vi "Create and Start gRPC Server.vi"(5 "Server Key File (.key)":path, 7 "Server Certificate File (.crt)":path, 8 "error in (no error)":errorcluster, 10 "Server Address":string="localhost:15882", 11 "Plugin Manager in":refnum<class "CIFPluginManager.lvclass">) -> (0 "error out":errorcluster, 3 "Plugin Manager out":refnum<class "CIFPluginManager.lvclass">)   [LabVIEW 2021, in "CIFPluginManager.lvclass"]
uses:
  CIFPluginManager.lvclass
  <vilib>/gRPC/LabVIEW gRPC Servicer/Servicer/Servicer.lvclass/Servicer.ctl
  CIFPluginManager.lvclass/CIFPluginManager.ctl
  <vilib>/gRPC/LabVIEW gRPC Servicer/Servicer/Servicer.lvclass
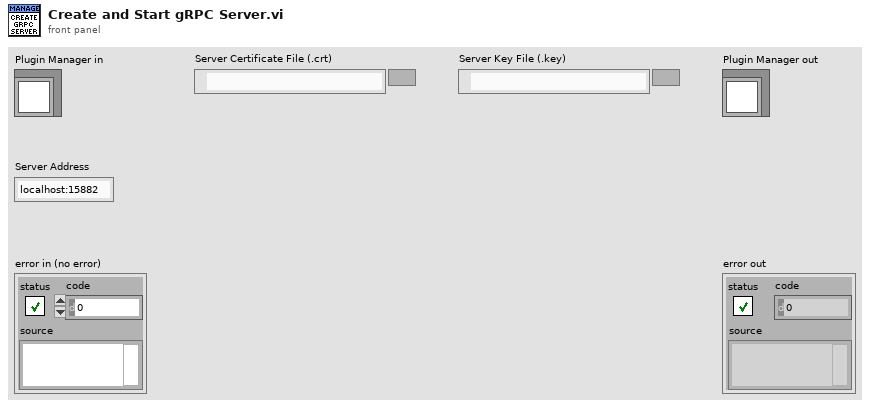
[diagram p1: front panel]
types:
  T1 = typedef "grpc-lvsupport-release.lvlib/grpcId.ctl" = u64
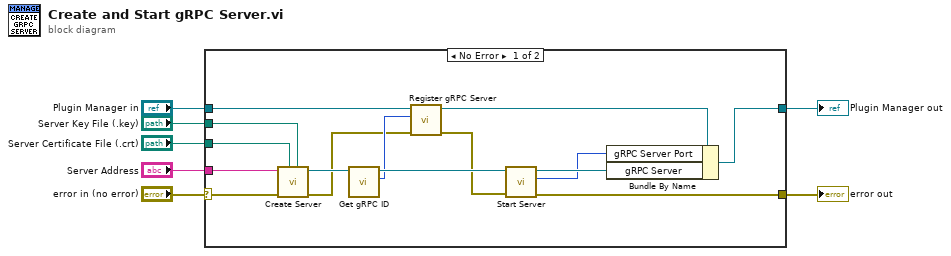
[diagram p0: block diagram]
diagram:
  n1 = case shown="No Error" "error in (no error)" {
    selector: "error in (no error)" -> [w18 w24]
    tunnel: [w14 w24] -> w2
    tunnel: [w11 w23] -> w6
    tunnel: "Plugin Manager in" -> [w17 w23]
    tunnel: "Server Certificate File (.crt)" -> [w20 _]
    tunnel: "Server Key File (.key)" -> [w19 _]
    tunnel: "Server Address" -> [w8 _]
    frame No Error {
      n2 = call <vilib>:"Create Server.vi"("Server Key File (.key)"=w19, "Server Certificate File (.crt)"=w20, "error in"=w18, "Server Address"=w8) -> ("error out"=w15:errorcluster, "gRPC Server out"=w22:refnum<class "Servicer.lvclass">)  [unwired: 6 in]
      n3 = call <vilib>:"Get gRPC ID.vi"("OOP Server in"=w22) -> ("gRPC ID"=w16:T1, "OOP Server out"=w21:refnum<class "Servicer.lvclass">)  [unwired: 9 in]
      n4 = call "Register gRPC Server.vi"("error in (no error)"=w15, "gRPC ID"=w16, "Plugin Manager in"=w17) -> ("error out"=w9:errorcluster, "Plugin Manager out"=w10:refnum<class "CIFPluginManager.lvclass">)  [unwired: 7 in]
      n5 = call <vilib>:"Start Server.vi"("error in"=w9, "gRPC Server in"=w21) -> ("error out"=w14:errorcluster, "Listening Port"=w12:i32, "gRPC Server out"=w13:refnum<class "Servicer.lvclass">)  [unwired: 7 in]
      n6 = Bundle By Name(cluster=w10, "gRPC Server Port"=w12, "gRPC Server"=w13) -> (w11:refnum<class "CIFPluginManager.lvclass">)
    }
    frame Error {
    }
  }
  "error out" <- w2
  "Plugin Manager out" <- w6
